vi "mxwScript_API_Option_UseLabVIEWSpecificTemplatePaths.vi"(0 "options in":T2[](array[typedef]), 1 "pathGenerationType":T1, 5 "locationIndex":u32, 7 "locationName":string, 9 "pathFormat":string, 11 "error in (no error)":errorcluster, 12 "useLVVersionIncrement":bool) -> (4 "options out":T2[](array[typedef]), 15 "error out":errorcluster)   [LabVIEW 2020]
doc: "Sets whether or not to use LabVIEW version specific template paths. This is useful if you are generating code to multiple versions of LabVIEW and need to specify which template set to use."
uses:
  codeGenAPISupport.llb/cgAPI_mxwScript_OptionData.ctl
  mxwScript_Option_LVSpecificTemplPathsGenType.ctl
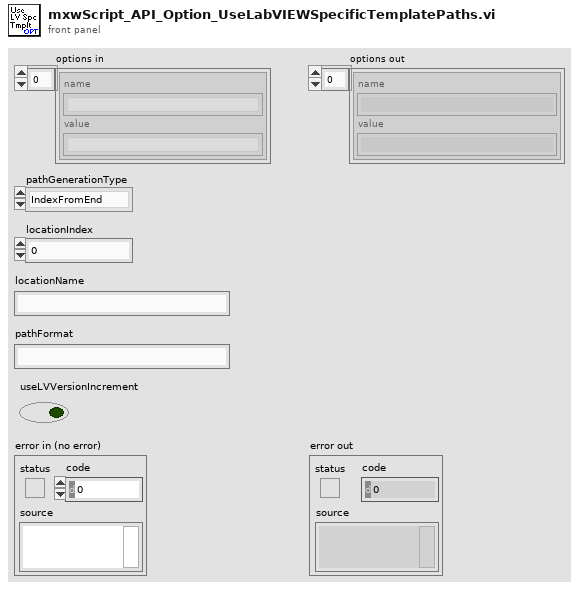
[diagram p1: front panel]
types:
  T1 = typedef "mxwScript_Option_LVSpecificTemplPathsGenType.ctl" = enum16{"IndexFromEnd", "Name", "BeforeLLB"}
  T2 = typedef "cgAPI_mxwScript_OptionData.ctl" = cluster{"name":string, "value":string}
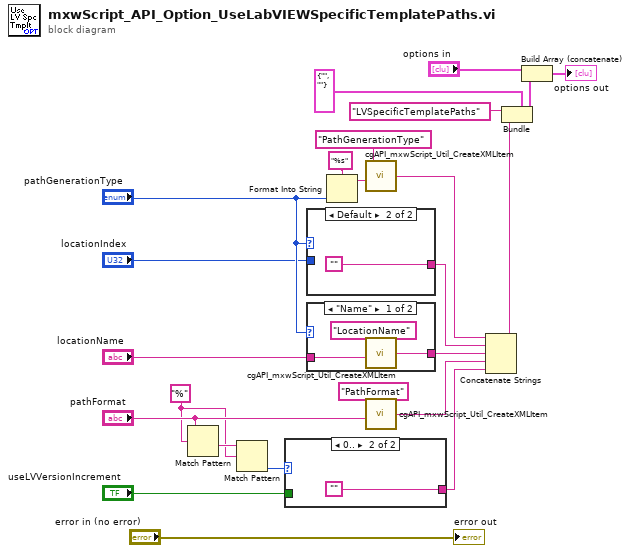
[diagram p0: block diagram]
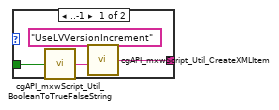
[diagram p2: hidden frame]
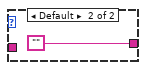
[diagram p3: hidden frame]
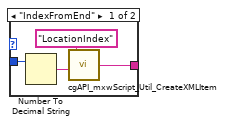
[diagram p4: hidden frame]
diagram:
  w2 = "%" ("regular expression")
  n1 = Match Pattern(string="pathFormat", regular expression=w2) -> (after substring=w3:string)  [unwired: 4 out]
  n2 = Match Pattern(string=w3, regular expression=w2) -> (offset past match=w1:i32)  [unwired: 4 out]
  n3 = case shown="0.." w1 {
    tunnel: "useLVVersionIncrement" -> [w25 _]
    tunnel: [w27 ""] -> w14
    frame ..-1 {
      n4 = call "cgAPI_mxwScript_Util_BooleanToTrueFalseString.vi"("boolean"=w25) -> ("TRUE/FALSE text"=w26:string)  [unwired: 4 out]
      n5 = call "cgAPI_mxwScript_Util_CreateXMLItem.vi"("value"=w26, "tag"="UseLVVersionIncrement") -> ("item"=w27:string)  [unwired: 4 out]
    }
    frame 0.. {
    }
  }
  n6 = case shown="Default" "pathGenerationType" {
    tunnel: "locationIndex" -> [w31 _]
    tunnel: [w32 ""] -> w17
    frame "IndexFromEnd" {
      n7 = Number To Decimal String(number=w31) -> (decimal integer string=w30:string)  [unwired: 1 out]
      n8 = call "cgAPI_mxwScript_Util_CreateXMLItem.vi"("value"=w30, "tag"="LocationIndex") -> ("item"=w32:string)  [unwired: 4 out]
    }
    frame Default {
    }
  }
  n9 = case shown="\"Name\"" "pathGenerationType" {
    tunnel: "locationName" -> [w35 _]
    tunnel: [w36 ""] -> w16
    frame "Name" {
      n10 = call "cgAPI_mxwScript_Util_CreateXMLItem.vi"("value"=w35, "tag"="LocationName") -> ("item"=w36:string)  [unwired: 4 out]
    }
    frame Default {
    }
  }
  n11 = Format Into String(format string="%s", "pathGenerationType") -> (resulting string=w6:string)  [unwired: 2 in, 1 out]
  n12 = call "cgAPI_mxwScript_Util_CreateXMLItem.vi"("value"=w6, "tag"="PathGenerationType") -> ("item"=w18:string)  [unwired: 4 out]
  n13 = call "cgAPI_mxwScript_Util_CreateXMLItem.vi"("value"="pathFormat", "tag"="PathFormat") -> ("item"=w15:string)  [unwired: 4 out]
  n14 = Concatenate Strings(w18, w17, w16, w15, w14) -> (w13:string)
  n15 = Bundle(cluster=T2 {"name"="", "value"=""} ("optionData"), "name"="LVSpecificTemplatePaths", "value"=w13) -> (w22:T2)
  n16 = Build Array (concatenate)("options in", w22) -> (→"options out":T2[])
  "error out" <- "error in (no error)"
